vi "Count Times Data Increases in Value.vi"(1 "Data":i32[](array[numeric])) -> (0 "Count Increases":i32)   [LabVIEW 2020, in "Advent of Code.lvlib"]
uses:
  Advent of Code.lvlib
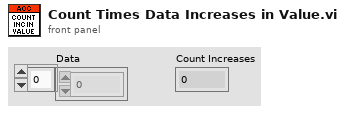
[diagram p1: front panel]
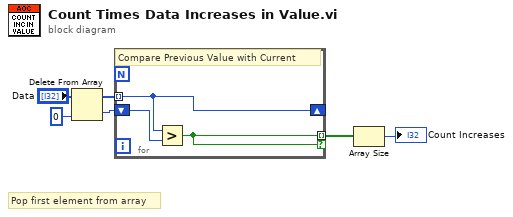
[diagram p0: block diagram]
diagram:
  # "Pop first element from array"
  n1 = Delete From Array(array="Data", index=0) -> (deleted portion=w4:i32, array with subset deleted=w3:i32[])  [unwired: 1 in]
  n2 = for {
    tunnel: w3 -> [w8] mode=indexing
    shift-right: [w8] -> _
    shift-left: w4 -> [w9]
    tunnel: [w7] -> w5 mode=indexing if=w7
    # "Compare Previous Value with Current"
    n3 = Greater?(x=w8, y=w9) -> (0:w7:bool)
  }
  n4 = Array Size(array=w5) -> (size(s)=→"Count Increases":i32)
